vi "BRig_RT_panel_cue_v1,18.vi"(7 "input_setValues":bool, 11 "input_dataExp":u16[](array[numeric])) -> (3 "output_dataExp":u16[](array[numeric]))   [LabVIEW 2014]
panel:
  in  "Cue2_1A_LorR":bool
  in  "Cue2_1A_Prob":u16
  in  "sp__Cue1B":u16(slide)=2 max=2 step=1 scale=0.0..2.0
  in  "Audio_Amp__Cue1B":u16=100 caption="Amp"
  in  "Audio_Freq__Cue1B":u16=5 caption="Freq [kHz]" max=14 step=1
  in  "CueLed_baseline":bool
  in  "CueSwitch_Count_PostR":u16
  in  "CueSwitch_Prob_PostR":u16
  in  "CueSwitch_PostR":u16(slide) max=3 step=1 scale=0.0..3.0
  in  "CueSwitch_Count_PreR":u16
  in  "CueSwitch_Count_First":u16
  in  "CueSwitch_Prob_PreR":u16
  in  "CueSwitch_PreR":u16(slide) max=3 step=1 scale=0.0..3.0
  in  "CueSwitch_Prob_First":u16
  in  "CueSwitch_First":u16(slide) max=3 step=1 scale=0.0..3.0
  in  "CueLed_Freq":u16=10
  in  "CueLed_Tpeak":u16=2
  in  "sp_RightSpout":u16(slide)=2 max=2 step=1 scale=0.0..2.0
  in  "sp_LeftSpout":u16(slide)=2 max=2 step=1 scale=0.0..2.0
  in  "Audio_Amp__R":u16=100 caption="Amp"
  in  "Audio_Freq__R":u16=5 caption="Freq [kHz]" max=14 step=1
  in  "Audio_Amp__L":u16=100 caption="Amp"
  in  "Audio_Freq__L":u16=5 caption="Freq [kHz]" max=14 step=1
  # "Cue State\n                                             Cue Type         LED Probability    Count"
  # "Audio or LED"
  # "First"
  # "Pre Reward"
  # "Post Reward"
  # "Audio Parameters"
  # "Cue LED Parameters"
  # "Left                  Right"
  # "Frequency\n[Hz]"
  # "Frequency\n[kHz]"
  # "1A\n1B"
  # "2"
  # "Timing [ms]\n                    Peak Width"
  # "Amp\n(0 - 32,000)"
  # "1A\n1B"
  # "2"
  # "1A  1B"
  # "2"
  # "Speaker\nPattern\nDuring Cue"
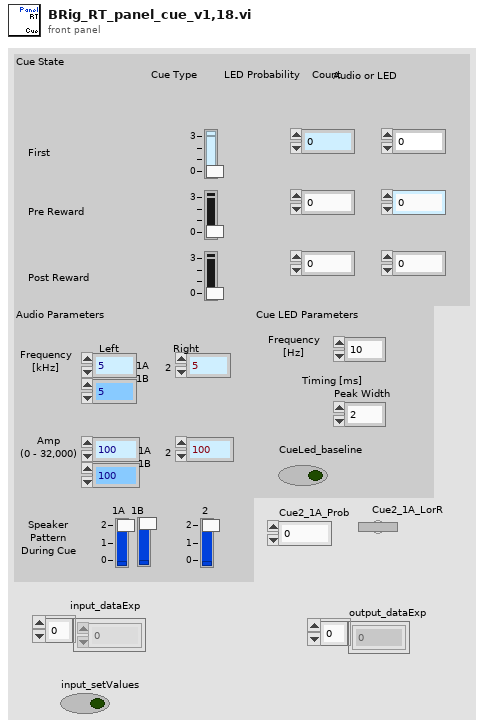
[diagram p1: front panel]
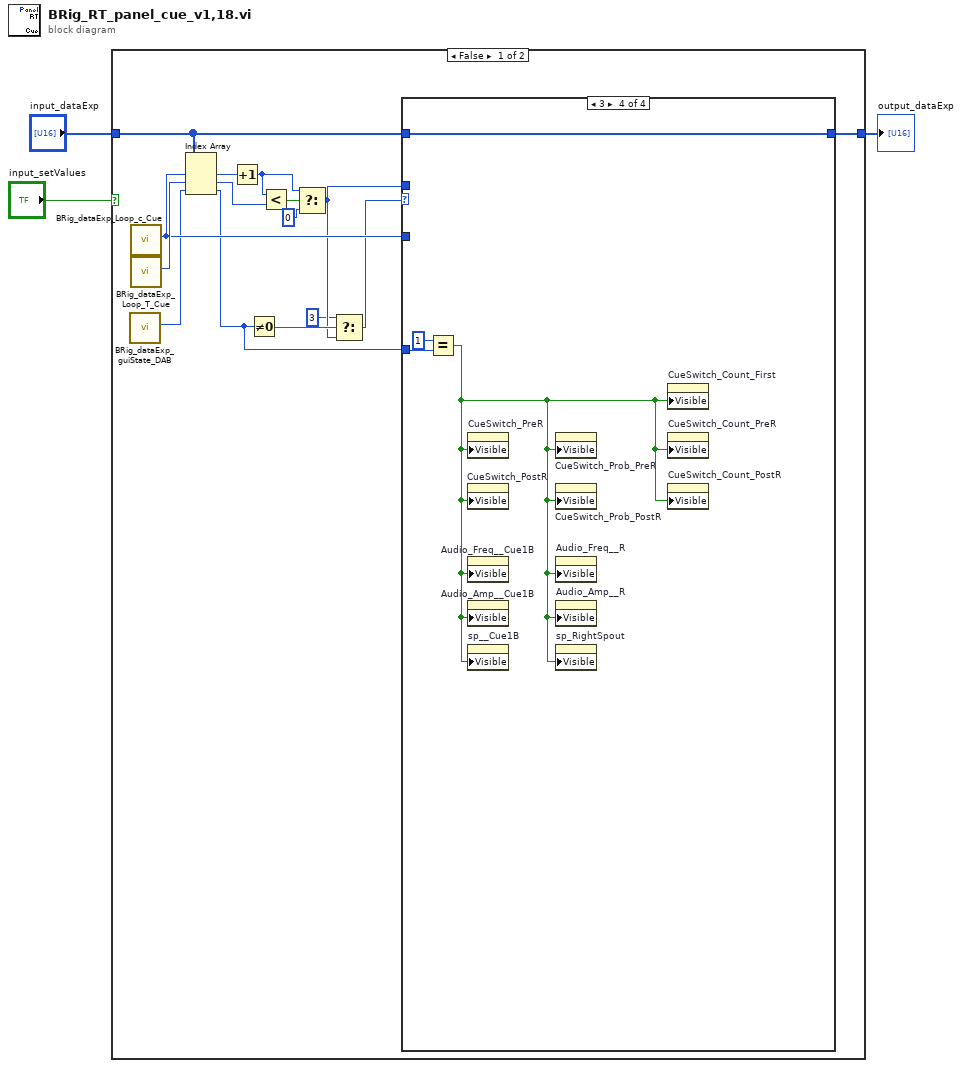
[diagram p0: block diagram]
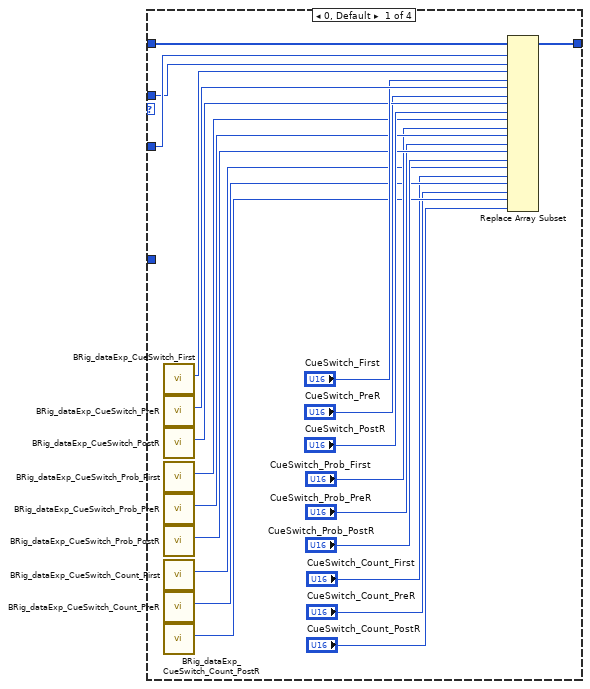
[diagram p2: hidden frame]
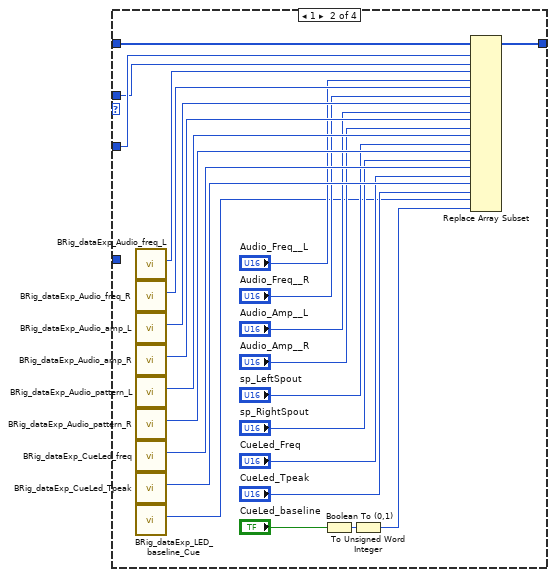
[diagram p3: hidden frame]
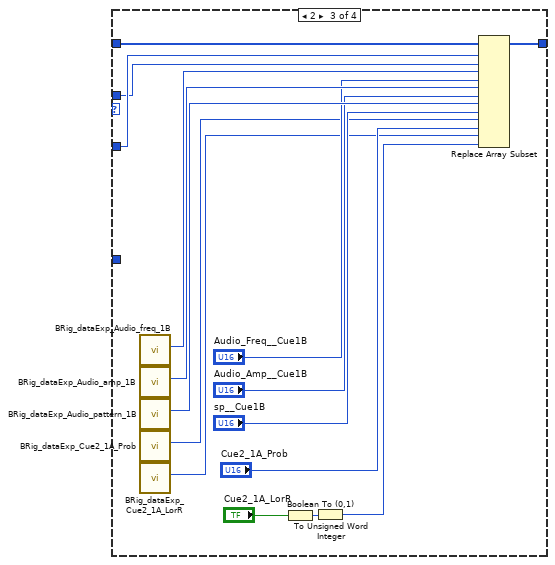
[diagram p4: hidden frame]
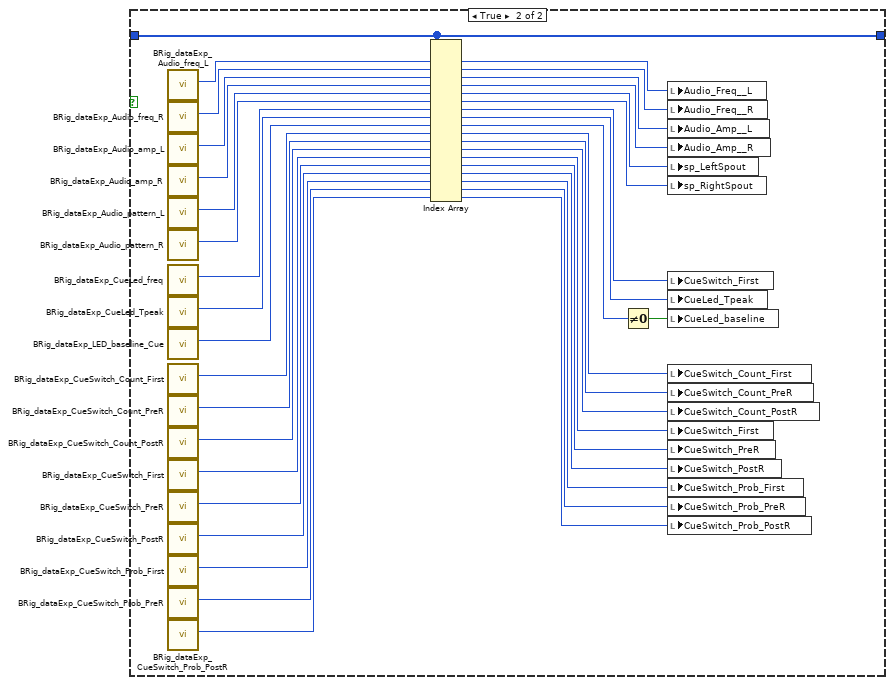
[diagram p5: hidden frame]
diagram:
  n1 = case shown="False" "input_setValues" {
    tunnel: "input_dataExp" -> [w13 w122]
    tunnel: [w12 w122] -> w2
    frame False {
      n2 = call "BRig_dataExp_guiState_DAB.vi"() -> ("output_guiState_DAB"=w10:i32)  [unwired: 11 in]
      n3 = call "BRig_dataExp_Loop_c_Cue.vi"() -> ("output_Loop_c_Cue"=w11:i32)  [unwired: 11 in]
      n4 = call "BRig_dataExp_Loop_T_Cue.vi"() -> ("output_Loop_T_Cue"=w18:i32)  [unwired: 11 in]
      n5 = Index Array(array=w13, index #1=w11, index #2=w18, index #3=w10) -> (element #1=w17:u16, element #2=w5:u16, element #3=w4:u16)
      n6 = Increment(x=w17) -> (x+1=w15:u16)
      n7 = Not Equal To 0?(x=w4) -> (x != 0?=w9:bool)
      n8 = Less?(x=w15, y=w5) -> (x < y?=w16:bool)
      n9 = Select(t=w15, s=w16, f=u16 0) -> (s? t:f=w8:u16)
      n10 = Select(t=u16 3, s=w9, f=w8) -> (s? t:f=w6:u16)
      n11 = case shown="3" w6 {
        tunnel: w13 -> [w40 w64 w80 w84]
        tunnel: [w21 w63 w79 w84] -> w12
        tunnel: w11 -> [w20 w62 w66 _]
        tunnel: w8 -> [w19 w61 w65 _]
        tunnel: w4 -> [_ _ _ w83]
        frame 0, Default {
          n12 = call "BRig_dataExp_CueSwitch_First.vi"() -> ("output_CueSwitch_First"=w39:i32)  [unwired: 11 in]
          n13 = call "BRig_dataExp_CueSwitch_PreR.vi"() -> ("output_CueSwitch_PreR"=w38:i32)  [unwired: 11 in]
          n14 = call "BRig_dataExp_CueSwitch_PostR.vi"() -> ("output_CueSwitch_PostR"=w36:i32)  [unwired: 11 in]
          n15 = call "BRig_dataExp_CueSwitch_Prob_First.vi"() -> ("output_CueSwitch_Prob_First"=w33:i32)  [unwired: 11 in]
          n16 = call "BRig_dataExp_CueSwitch_Prob_PreR.vi"() -> ("output_CueSwitch_Prob_PreR"=w32:i32)  [unwired: 11 in]
          n17 = call "BRig_dataExp_CueSwitch_Prob_PostR.vi"() -> ("output_CueSwitch_Prob_PostR"=w31:i32)  [unwired: 11 in]
          n18 = call "BRig_dataExp_CueSwitch_Count_First.vi"() -> ("output_CueSwitch_Count_First"=w27:i32)  [unwired: 11 in]
          n19 = call "BRig_dataExp_CueSwitch_Count_PreR.vi"() -> ("output_CueSwitch_Count_PreR"=w26:i32)  [unwired: 11 in]
          n20 = call "BRig_dataExp_CueSwitch_Count_PostR.vi"() -> ("output_CueSwitch_Count_PostR"=w25:i32)  [unwired: 11 in]
          n21 = Replace Array Subset(array=w40, new element #1=w19, index #1=w20, new element #2="CueSwitch_First", index #2=w39, new element #3="CueSwitch_PreR", index #3=w38, new element #4="CueSwitch_PostR", index #4=w36, new element #5="CueSwitch_Prob_First", index #5=w33, new element #6="CueSwitch_Prob_PreR", index #6=w32, new element #7="CueSwitch_Prob_PostR", index #7=w31, new element #8="CueSwitch_Count_First", index #8=w27, new element #9="CueSwitch_Count_PreR", index #9=w26, new element #10="CueSwitch_Count_PostR", index #10=w25) -> (w21:u16[])
        }
        frame 1 {
          n22 = call "BRig_dataExp_Audio_freq_L.vi"() -> ("output_Audio_freq__L"=w60:i32)  [unwired: 11 in]
          n23 = call "BRig_dataExp_Audio_freq_R.vi"() -> ("output_Audio_freq__R"=w59:i32)  [unwired: 11 in]
          n24 = call "BRig_dataExp_Audio_amp_L.vi"() -> ("output_Audio_amp__L"=w58:i32)  [unwired: 11 in]
          n25 = call "BRig_dataExp_Audio_amp_R.vi"() -> ("output_Audio_amp__R"=w57:i32)  [unwired: 11 in]
          n26 = call "BRig_dataExp_Audio_pattern_L.vi"() -> ("output_Audio_sp__L"=w56:i32)  [unwired: 11 in]
          n27 = call "BRig_dataExp_Audio_pattern_R.vi"() -> ("output_Audio_sp__R"=w55:i32)  [unwired: 11 in]
          n28 = call "BRig_dataExp_CueLed_freq.vi"() -> ("output_CueLed_Freq"=w54:i32)  [unwired: 11 in]
          n29 = call "BRig_dataExp_CueLed_Tpeak.vi"() -> ("output_CueLed_Tpeak"=w53:i32)  [unwired: 11 in]
          n30 = call "BRig_dataExp_LED_baseline_Cue.vi"() -> ("output_LED_baseline_Cue"=w44:i32)  [unwired: 11 in]
          n31 = Boolean To (0,1)(Boolean="CueLed_baseline") -> (0, 1=w42:i16)
          n32 = To Unsigned Word Integer(number=w42) -> (unsigned 16bit integer=w41:u16)
          n33 = Replace Array Subset(array=w64, new element #1=w61, index #1=w62, new element #2="Audio_Freq__L", index #2=w60, new element #3="Audio_Freq__R", index #3=w59, new element #4="Audio_Amp__L", index #4=w58, new element #5="Audio_Amp__R", index #5=w57, new element #6="sp_LeftSpout", index #6=w56, new element #7="sp_RightSpout", index #7=w55, new element #8="CueLed_Freq", index #8=w54, new element #9="CueLed_Tpeak", index #9=w53, new element #10=w41, index #10=w44) -> (w63:u16[])
        }
        frame 2 {
          n34 = call "BRig_dataExp_Audio_freq_1B.vi"() -> ("output_Audio_freq__1B"=w78:i32)  [unwired: 11 in]
          n35 = call "BRig_dataExp_Audio_amp_1B.vi"() -> ("output_Audio_amp__1B"=w77:i32)  [unwired: 11 in]
          n36 = call "BRig_dataExp_Audio_pattern_1B.vi"() -> ("output_Audio_sp__1B"=w76:i32)  [unwired: 11 in]
          n37 = call "BRig_dataExp_Cue2_1A_Prob.vi"() -> ("output_Cue2_1A_Prob"=w72:i32)  [unwired: 11 in]
          n38 = call "BRig_dataExp_Cue2_1A_LorR.vi"() -> ("output_Cue2_1A_LorR"=w70:i32)  [unwired: 11 in]
          n39 = Boolean To (0,1)(Boolean="Cue2_1A_LorR") -> (0, 1=w68:i16)
          n40 = To Unsigned Word Integer(number=w68) -> (unsigned 16bit integer=w67:u16)
          n41 = Replace Array Subset(array=w80, new element #1=w65, index #1=w66, new element #2="Audio_Freq__Cue1B", index #2=w78, new element #3="Audio_Amp__Cue1B", index #3=w77, new element #4="sp__Cue1B", index #4=w76, new element #5="Cue2_1A_Prob", index #5=w72, new element #6=w67, index #6=w70) -> (w79:u16[])
        }
        frame 3 {
          n42 = Equal?(x=u16 1, y=w83) -> (x = y?=w81:bool)
          n43 = property on="CueSwitch_PreR" class="Slide (strict)"("Visible"=w81) -> ()  [unwired: 2 in, 2 out]
          n44 = property on="CueSwitch_PostR" class="Slide (strict)"("Visible"=w81) -> ()  [unwired: 2 in, 2 out]
          n45 = property on="Audio_Freq__Cue1B" class="DigNum (strict)"("Visible"=w81) -> ()  [unwired: 2 in, 2 out]
          n46 = property on="Audio_Amp__Cue1B" class="DigNum (strict)"("Visible"=w81) -> ()  [unwired: 2 in, 2 out]
          n47 = property on="sp__Cue1B" class="Slide (strict)"("Visible"=w81) -> ()  [unwired: 2 in, 2 out]
          n48 = property on="CueSwitch_Prob_PreR" class="DigNum (strict)"("Visible"=w81) -> ()  [unwired: 2 in, 2 out]
          n49 = property on="CueSwitch_Prob_PostR" class="DigNum (strict)"("Visible"=w81) -> ()  [unwired: 2 in, 2 out]
          n50 = property on="Audio_Freq__R" class="DigNum (strict)"("Visible"=w81) -> ()  [unwired: 2 in, 2 out]
          n51 = property on="Audio_Amp__R" class="DigNum (strict)"("Visible"=w81) -> ()  [unwired: 2 in, 2 out]
          n52 = property on="sp_RightSpout" class="Slide (strict)"("Visible"=w81) -> ()  [unwired: 2 in, 2 out]
          n53 = property on="CueSwitch_Count_First" class="DigNum (strict)"("Visible"=w81) -> ()  [unwired: 2 in, 2 out]
          n54 = property on="CueSwitch_Count_PreR" class="DigNum (strict)"("Visible"=w81) -> ()  [unwired: 2 in, 2 out]
          n55 = property on="CueSwitch_Count_PostR" class="DigNum (strict)"("Visible"=w81) -> ()  [unwired: 2 in, 2 out]
        }
      }
    }
    frame True {
      n56 = call "BRig_dataExp_Audio_freq_L.vi"() -> ("output_Audio_freq__L"=w121:i32)  [unwired: 11 in]
      n57 = call "BRig_dataExp_Audio_freq_R.vi"() -> ("output_Audio_freq__R"=w119:i32)  [unwired: 11 in]
      n58 = call "BRig_dataExp_Audio_amp_L.vi"() -> ("output_Audio_amp__L"=w117:i32)  [unwired: 11 in]
      n59 = call "BRig_dataExp_Audio_amp_R.vi"() -> ("output_Audio_amp__R"=w115:i32)  [unwired: 11 in]
      n60 = call "BRig_dataExp_Audio_pattern_L.vi"() -> ("output_Audio_sp__L"=w113:i32)  [unwired: 11 in]
      n61 = call "BRig_dataExp_Audio_pattern_R.vi"() -> ("output_Audio_sp__R"=w112:i32)  [unwired: 11 in]
      n62 = call "BRig_dataExp_CueLed_freq.vi"() -> ("output_CueLed_Freq"=w109:i32)  [unwired: 11 in]
      n63 = call "BRig_dataExp_CueLed_Tpeak.vi"() -> ("output_CueLed_Tpeak"=w107:i32)  [unwired: 11 in]
      n64 = call "BRig_dataExp_LED_baseline_Cue.vi"() -> ("output_LED_baseline_Cue"=w105:i32)  [unwired: 11 in]
      n65 = call "BRig_dataExp_CueSwitch_Count_First.vi"() -> ("output_CueSwitch_Count_First"=w102:i32)  [unwired: 11 in]
      n66 = call "BRig_dataExp_CueSwitch_Count_PreR.vi"() -> ("output_CueSwitch_Count_PreR"=w101:i32)  [unwired: 11 in]
      n67 = call "BRig_dataExp_CueSwitch_Count_PostR.vi"() -> ("output_CueSwitch_Count_PostR"=w100:i32)  [unwired: 11 in]
      n68 = call "BRig_dataExp_CueSwitch_First.vi"() -> ("output_CueSwitch_First"=w99:i32)  [unwired: 11 in]
      n69 = call "BRig_dataExp_CueSwitch_PreR.vi"() -> ("output_CueSwitch_PreR"=w98:i32)  [unwired: 11 in]
      n70 = call "BRig_dataExp_CueSwitch_PostR.vi"() -> ("output_CueSwitch_PostR"=w97:i32)  [unwired: 11 in]
      n71 = call "BRig_dataExp_CueSwitch_Prob_First.vi"() -> ("output_CueSwitch_Prob_First"=w96:i32)  [unwired: 11 in]
      n72 = call "BRig_dataExp_CueSwitch_Prob_PreR.vi"() -> ("output_CueSwitch_Prob_PreR"=w95:i32)  [unwired: 11 in]
      n73 = call "BRig_dataExp_CueSwitch_Prob_PostR.vi"() -> ("output_CueSwitch_Prob_PostR"=w94:i32)  [unwired: 11 in]
      n74 = Index Array(array=w122, index #1=w121, index #2=w119, index #3=w117, index #4=w115, index #5=w113, index #6=w112, index #7=w109, index #8=w107, index #9=w105, index #10=w102, index #11=w101, index #12=w100, index #13=w99, index #14=w98, index #15=w97, index #16=w96, index #17=w95, index #18=w94) -> (element #1=w120:u16, element #2=w118:u16, element #3=w116:u16, element #4=w114:u16, element #5=w111:u16, element #6=w110:u16, element #7=w108:u16, element #8=w106:u16, element #9=w103:u16, element #10=w93:u16, element #11=w92:u16, element #12=w91:u16, element #13=w90:u16, element #14=w89:u16, element #15=w88:u16, element #16=w87:u16, element #17=w86:u16, element #18=w85:u16)
      n75 = Not Equal To 0?(x=w103) -> (x != 0?=w104:bool)
      n76 = local write "Audio_Freq__L"(w120) -> ()
      n77 = local write "Audio_Freq__R"(w118) -> ()
      n78 = local write "Audio_Amp__L"(w116) -> ()
      n79 = local write "Audio_Amp__R"(w114) -> ()
      n80 = local write "sp_LeftSpout"(w111) -> ()
      n81 = local write "sp_RightSpout"(w110) -> ()
      n82 = local write "CueSwitch_First"(w108) -> ()
      n83 = local write "CueLed_Tpeak"(w106) -> ()
      n84 = local write "CueLed_baseline"(w104) -> ()
      n85 = local write "CueSwitch_Count_First"(w93) -> ()
      n86 = local write "CueSwitch_Count_PreR"(w92) -> ()
      n87 = local write "CueSwitch_Count_PostR"(w91) -> ()
      n88 = local write "CueSwitch_First"(w90) -> ()
      n89 = local write "CueSwitch_PreR"(w89) -> ()
      n90 = local write "CueSwitch_PostR"(w88) -> ()
      n91 = local write "CueSwitch_Prob_First"(w87) -> ()
      n92 = local write "CueSwitch_Prob_PreR"(w86) -> ()
      n93 = local write "CueSwitch_Prob_PostR"(w85) -> ()
    }
  }
  "output_dataExp" <- w2
